vi "Is Type.vi"(10 "Type":refnum<class "Value.lvclass">, 11 "Value":refnum<class "Value.lvclass">) -> (3 "Type Matches":bool)   [LabVIEW 2020, in "Promises.lvlib" / "Value.lvclass"]
uses:
  Value.lvclass
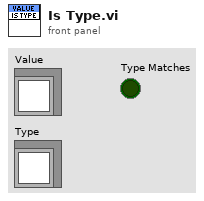
[diagram p1: front panel]
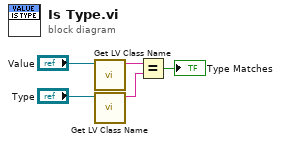
[diagram p0: block diagram]
diagram:
  n1 = call <vilib>:"Get LV Class Name.vi"("object"="Value") -> ("class name"=w5:string)  [unwired: 9 in, 1 out]
  n2 = call <vilib>:"Get LV Class Name.vi"("object"="Type") -> ("class name"=w4:string)  [unwired: 9 in, 1 out]
  n3 = Equal?(x=w5, y=w4) -> (x = y?=→"Type Matches":bool)
